vi "homework2.vi"() -> ()   [LabVIEW 2017]
panel:
  out "ans":dbl[](array[numeric])
  out "后五个元素":dbl[](array[numeric])
  out "前五个元素":dbl[](array[numeric])
  out "颠倒数组":dbl[](array[numeric])
  out "原始数组":dbl[](array[numeric])
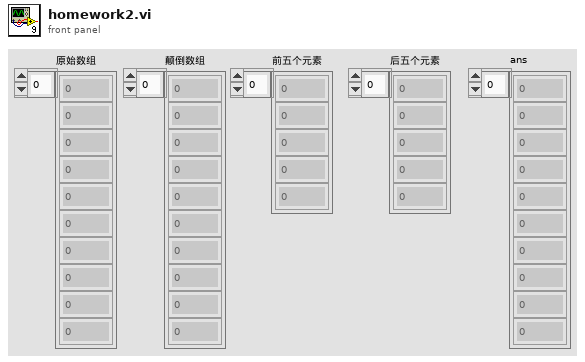
[diagram p1: front panel]
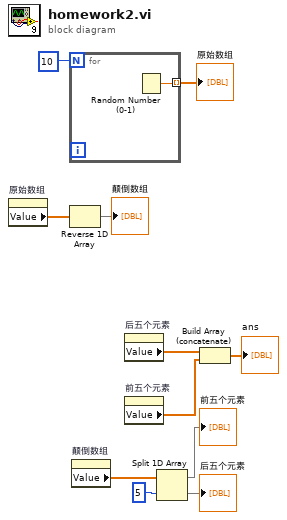
[diagram p0: block diagram]
diagram:
  n1 = property on="原始数组" class="Arr (严格)"() -> ("Value"=w9:dbl[])  [unwired: 2 in, 2 out]
  n2 = for {
    N: 10 -> [_]
    tunnel: [w12] -> w10 mode=indexing
    n3 = Random Number (0-1)() -> (number: 0 to 1=w12:dbl)
  }
  "原始数组" <- w10
  n4 = Reverse 1D Array(array=w9) -> (reversed array=→"颠倒数组":dbl[])
  n5 = property on="颠倒数组" class="Arr (严格)"() -> ("Value"=w7:dbl[])  [unwired: 2 in, 2 out]
  n6 = property on="后五个元素" class="Arr (严格)"() -> ("Value"=w2:dbl[])  [unwired: 2 in, 2 out]
  n7 = property on="前五个元素" class="Arr (严格)"() -> ("Value"=w3:dbl[])  [unwired: 2 in, 2 out]
  n8 = Split 1D Array(array=w7, index=5 ("索引")) -> (first subarray=→"前五个元素":dbl[], second subarray=→"后五个元素":dbl[])
  n9 = Build Array (concatenate)(w2, w3) -> (→"ans":dbl[])
